vi "FTW-TransferClient-DownloadBegin.vi"(0 "Transfer Client":refnum<k24>, 5 "Remote URI":string, 7 "Local Filepath":path, 11 "error in":errorcluster) -> (4 "Transfer Client out":refnum<k24>, 6 "Download Events":refnum<event-registration>, 15 "error out":errorcluster)   [LabVIEW 2015]
uses:
  FTW-TransferClient-TransferProgress.ctl
  FTW-TransferClient-TransferStatus.ctl
panel:
  # "Inputs"
  # "Outputs"
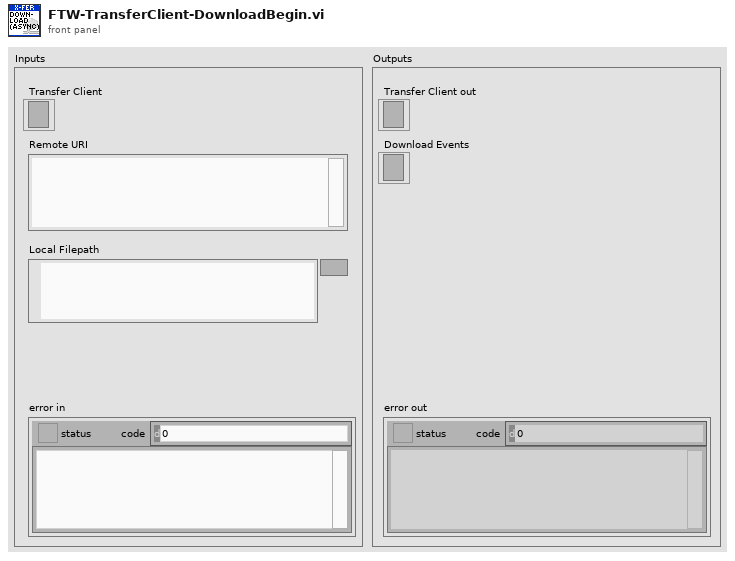
[diagram p1: front panel]
types:
  T1 = cluster{"Transfer Progress":refnum<user-event>, "Current Time":dbl, "AbsoluteURI":string, "Local Filepath":path}
  T2 = cluster{"Transfer Complete":refnum<user-event>, "Current Time":dbl, "AbsoluteURI":string, "Local Filepath":path}
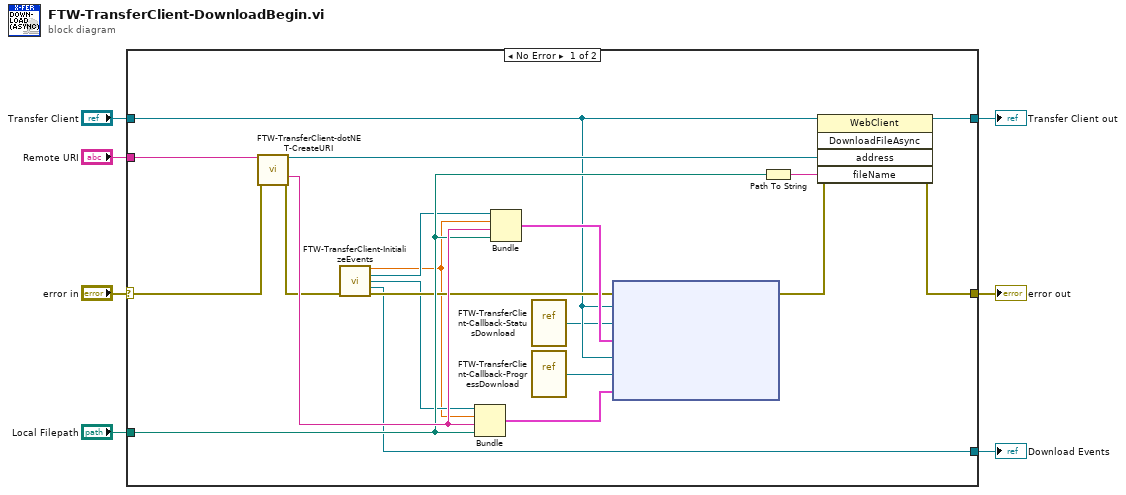
[diagram p0: block diagram]
diagram:
  n1 = case shown="No Error" "error in" {
    selector: "error in" -> [w23 w28]
    tunnel: "Transfer Client" -> [w10 w29]
    tunnel: [w20 w28] -> w7
    tunnel: [w9 w29] -> w6
    tunnel: "Local Filepath" -> [w24 _]
    tunnel: [w12 _] -> w2
    tunnel: "Remote URI" -> [w11 _]
    frame No Error {
      n2 = call "FTW-TransferClient-dotNET-CreateURI.vi"("URI"=w11, "error in"=w23) -> ("URI ref"=w26:refnum<k24>, "AbsoluteURI"=w25:string, "error out"=w17:errorcluster)  [unwired: 8 in, 3 out]
      n3 = call "FTW-TransferClient-InitializeEvents.vi"("error in"=w17) -> ("Current Time"=w13:dbl, "Transfer Complete"=w15:refnum<user-event>, "Transfer Progress"=w14:refnum<user-event>, "Transfer Events"=w12:refnum<event-registration>, "error out"=w16:errorcluster)  [unwired: 10 in]
      n4 = Bundle("Transfer Progress"=w14, "Current Time"=w13, "AbsoluteURI"=w25, "Local Filepath"=w24) -> (w22:T1)  [unwired: 1 in]
      n5 = Bundle("Transfer Complete"=w15, "Current Time"=w13, "AbsoluteURI"=w25, "Local Filepath"=w24) -> (w18:T2)  [unwired: 1 in]
      n6 = vi-ref "FTW-TransferClient-Callback-StatusDownload.vi"() -> ("vi reference"=w8:refnum<vi>)
      n7 = vi-ref "FTW-TransferClient-Callback-ProgressDownload.vi"() -> ("vi reference"=w19:refnum<vi>)
      n8 = node(w16, w10, w8, w18, w10, w19, w22) -> (w21:errorcluster)  [unwired: 1 in, 1 out]
      n9 = Path To String(path=w24) -> (string=w27:string)
      n10 = invoke class="WebClient" method="DownloadFileAsync"(reference=w10, error in=w21, "address"=w26, "fileName"=w27) -> (reference out=w9:refnum<k24>, error out=w20:errorcluster)  [unwired: 1 in, 3 out]
    }
    frame Error {
    }
  }
  "error out" <- w7
  "Transfer Client out" <- w6
  "Download Events" <- w2
